vi "MSG Raise Error.vi"(8 "error in":errorcluster, 10 "raised error":cluster{"stop?":bool, "cause":string}={"stop?"=FALSE, "cause"="Error"}) -> (0 "error out":errorcluster)   [LabVIEW 2020, in "Manager.lvlib"]
doc: "Send component-specific API message: ERROR"
uses:
  Manager.lvlib
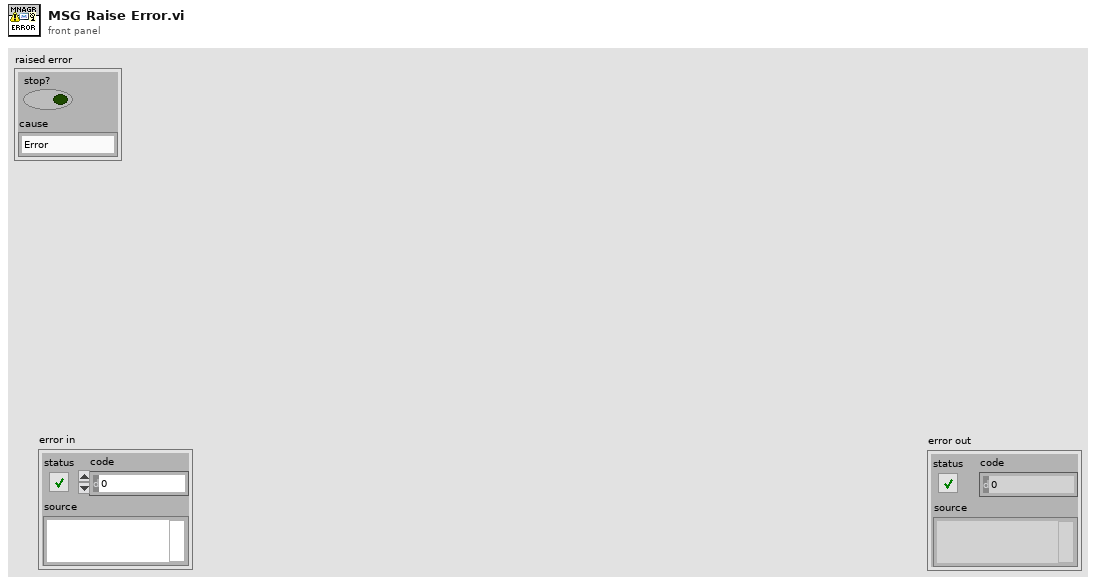
[diagram p1: front panel]
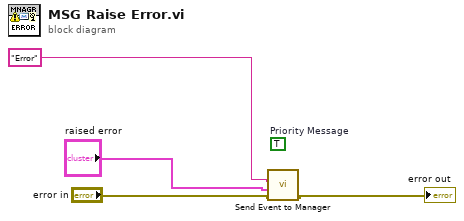
[diagram p0: block diagram]
diagram:
  (unwired) TRUE  # Priority Message
  n1 = call "Send Event to Manager.vi"("error in"="error in", "Payload"="raised error", "Command"="Error") -> ("error out"=→"error out":errorcluster)  [unwired: 8 in]
